vi "LEBITVacuum.PubSetServices.vi"(0 "i ref in":refnum<vi>, 2 "i attribute in":T1={"setValuePLC"=[], "nickNames"=[], "setValuePLCServiceID"=[], "monValuePLC"=[], "SetValueServiceID"=[], "MonValueServiceID"=[], "SetValue"=[], "AllPLCValues"=[], "CondSpecial2DArray"=[], "CondSpecialIndex"=[], "ReasonForLocking"="", "ReasonForLockingID"=0, "enableValuePLC"=[], "OverwriteCloseSafetyPLC"=[], "OverwriteOpenSafetyPLC"=[], "OverwriteCloseSafetyPLCServiceID"=[], "OverwriteOpenSafetyPLCServiceID"=[], "MKS Address Array"=[], "MKS MeasurementServiceID"=[], "MKS Measurement"=[], "CRYO Measurement"=[], "CRYO MeasurementServiceID"=[], "Special"=[], "Start Date"="", "MKS VISA resource"="COM13", "CRYO VISA resource"="COM13"}, 5 "error in":errorcluster) -> (14 "i ref out":refnum<vi>, 16 "i attribute out":T1={"setValuePLC"=[], "nickNames"=[], "setValuePLCServiceID"=[], "monValuePLC"=[], "SetValueServiceID"=[], "MonValueServiceID"=[], "SetValue"=[], "AllPLCValues"=[], "CondSpecial2DArray"=[], "CondSpecialIndex"=[], "ReasonForLocking"="", "ReasonForLockingID"=0, "enableValuePLC"=[], "OverwriteCloseSafetyPLC"=[], "OverwriteOpenSafetyPLC"=[], "OverwriteCloseSafetyPLCServiceID"=[], "OverwriteOpenSafetyPLCServiceID"=[], "MKS Address Array"=[], "MKS MeasurementServiceID"=[], "MKS Measurement"=[], "CRYO Measurement"=[], "CRYO MeasurementServiceID"=[], "Special"=[], "Start Date"="", "MKS VISA resource"="COM13", "CRYO VISA resource"="COM13"}, 17 "SetValueServiceID":i32[](array[numeric]), 19 "error out":errorcluster)   [LabVIEW 2014, in "LEBITVacuum.lvlib"]
uses:
  LEBITVacuum.lvlib
  CS_Core/CAEObj/CAEObj.event definition.ctl
  CS_Core/BaseProcess/BaseProcess.event definition.ctl
  CS_Core/BaseProcess/BaseProcess.descriptor string definition.ctl
  LEBITVacuum.i attribute.ctl
  CSlibraries/UtilityLib/UtilityLib.valueStatus.ctl
  CSlibraries/UtilityLib/UtilityLib.lvlib
  CS_Core/CSSystem/CoreLib/CoreLib.lvlib
  CSlibraries-extern/DimLVEvent/LVDimInterface/LVDimInterface.lvlib
  CS_Core/BaseProcess/BaseProcess.lvlib
  CS_Core/CAEObj/CAEObj.lvlib
panel:
  in  "event definition":T2
  in  "CAEEvtDef":T3
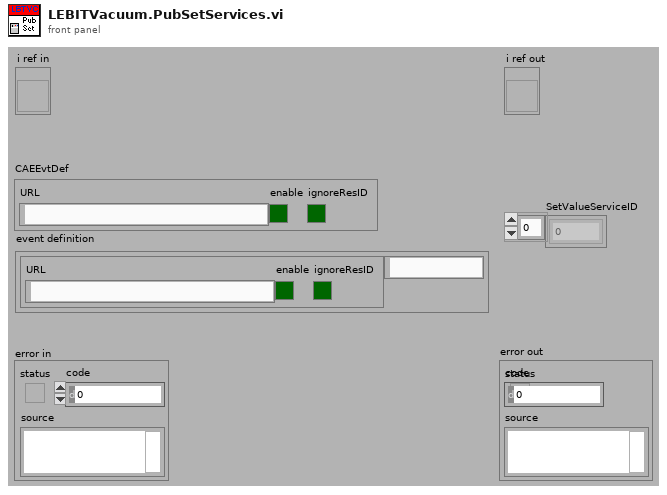
[diagram p1: front panel]
types:
  T1 = typedef "LEBITVacuum.lvlib/LEBITVacuum.i attribute.ctl" = cluster{"setValuePLC":string[], "nickNames":string[], "setValuePLCServiceID":i32[], "monValuePLC":string[], "SetValueServiceID":i32[], "MonValueServiceID":i32[], "SetValue":i16[], "AllPLCValues":string[], "CondSpecial2DArray":string[][], "CondSpecialIndex":i32[], "ReasonForLocking":string, "ReasonForLockingID":i32, "enableValuePLC":string[], "OverwriteCloseSafetyPLC":string[], "OverwriteOpenSafetyPLC":string[], "OverwriteCloseSafetyPLCServiceID":i32[], "OverwriteOpenSafetyPLCServiceID":i32[], "MKS Address Array":i32[][], "MKS MeasurementServiceID":i32[], "MKS Measurement":string[], "CRYO Measurement":string[][], "CRYO MeasurementServiceID":i32[], "Special":string[], "Start Date":string, "MKS VISA resource":refnum<visa-resource-name>, "CRYO VISA resource":refnum<visa-resource-name>}
  T2 = typedef "BaseProcess.lvlib/BaseProcess.event definition.ctl" = cluster{"CAEEvtDef":T3, "Data Descriptor":T4}
  T3 = typedef "CAEObj.lvlib/CAEObj.event definition.ctl" = cluster{"URL":string, "enable":bool, "ignoreResID":bool}
  T4 = typedef "BaseProcess.lvlib/BaseProcess.descriptor string definition.ctl" = string
  T5 = typedef "UtilityLib.lvlib/UtilityLib.valueStatus.ctl" = enum16{"no info available", "stand by/off", "on", "warning", "alarm/malfunction", "not implemented", "user action required", "important information", "system default", "control default", "indicator default", "button default"}
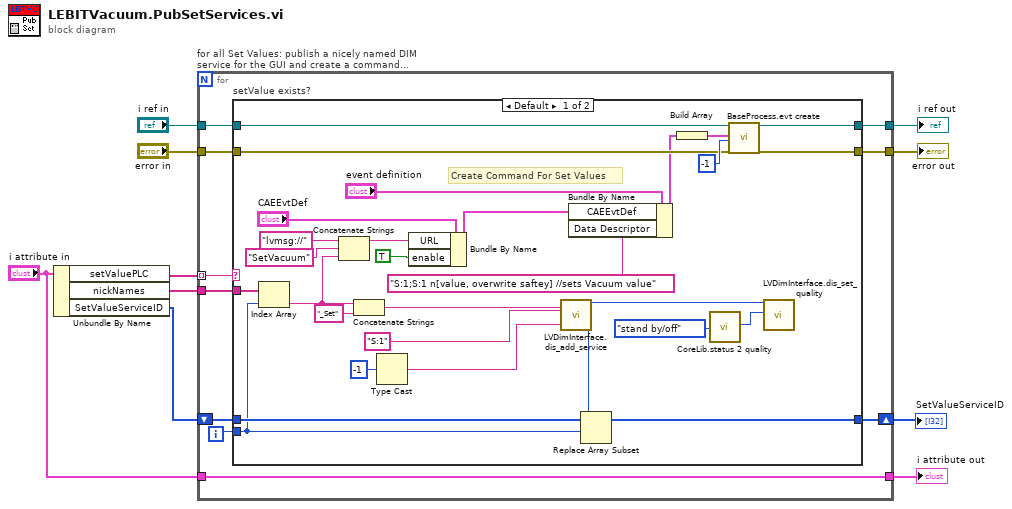
[diagram p0: block diagram]
diagram:
  n1 = Unbundle By Name("i attribute in") -> ("setValuePLC"=w4:string[], "nickNames"=w5:string[], "SetValueServiceID"=w1:i32[])
  n2 = for "for all Set Values: publish a nicely named DIM service for the GUI and create a command..." {
    tunnel: w4 -> [w20] mode=indexing
    tunnel: w5 -> [w19]
    shift-right: [w16] -> w10
    shift-left: w1 -> [w17]
    tunnel: "i ref in" -> [w15]
    tunnel: "error in" -> [w14]
    tunnel: [w13] -> w9
    tunnel: [w12] -> w8
    tunnel: "i attribute in" -> [w11]
    tunnel: [w11] -> w2
    i -> [w18]
    n3 = case "setValue exists?" shown="Default" w20 {
      tunnel: w19 -> [w46 _]
      tunnel: w18 -> [w27 _]
      tunnel: w17 -> [w44 w51]
      tunnel: [w43 w51] -> w16
      tunnel: w15 -> [w42 w50]
      tunnel: w14 -> [w24 w49]
      tunnel: [w32 w49] -> w13
      tunnel: [w31 w50] -> w12
      frame Default {
        # "Create Command For Set Values"
        n4 = Index Array(array=w46, index=w27) -> (element=w36:string)
        n5 = Concatenate Strings("lvmsg://" ("string"), "SetVacuum" ("string"), w36) -> (w39:string)
        n6 = Concatenate Strings(w36, "_Set" ("string")) -> (w47:string)
        n7 = Type Cast(x=i16 -1) -> (*(type *) &x=w45:string)  [unwired: 1 in]
        n8 = Bundle By Name(cluster="CAEEvtDef", "URL"=w39, "enable"=TRUE) -> (w40:T3)
        n9 = call "LVDimInterface.dis_add_service.vi"("serviceName"=w47, "typeDescriptor"="S:1", "data"=w45) -> ("my_serviceID"=w29:i32)  [unwired: 15 in, 1 out]
        n10 = Bundle By Name(cluster="event definition", "CAEEvtDef"=w40, "Data Descriptor"="S:1;S:1 n[value, overwrite saftey] //sets Vacuum value") -> (w23:T2)
        n11 = Replace Array Subset(array=w44, new element=w29, index=w27) -> (w43:i32[])
        n12 = Build Array(w23) -> (w33:T2[])
        n13 = call "CoreLib.status 2 quality.vi"("valueStatus"=UtilityLib.valueStatus."stand by/off") -> ("quality"=w28:i32)  [unwired: 18 in]
        n14 = call "BaseProcess.evt create.vi"("i ref in"=w42, "newEvents"=w33, "ms timeout (10000)"=-1, "error in (no error)"=w24) -> ("i ref out"=w31:refnum<vi>, "error out"=w32:errorcluster)  [unwired: 12 in, 2 out]
        n15 = call "LVDimInterface.dis_set_quality.vi"("my_serviceID"=w29, "quality"=w28) -> ()  [unwired: 16 in, 2 out]
      }
      frame "" {
      }
    }
  }
  "SetValueServiceID" <- w10
  "error out" <- w9
  "i ref out" <- w8
  "i attribute out" <- w2
